vi "Check for Target Crossing.vi"(7 "target value":dbl, 9 "previous value":dbl, 11 "current value":dbl) -> (3 "crossed":bool)   [LabVIEW 2022 SP3]
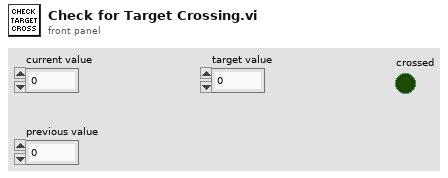
[diagram p1: front panel]
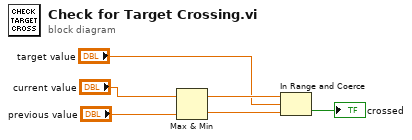
[diagram p0: block diagram]
diagram:
  n1 = Max & Min(x="current value", y="previous value") -> (max(x,y)=w6:dbl, min(x,y)=w5:dbl)
  n2 = In Range and Coerce(upper limit=w6, x="target value", lower limit=w5) -> (In Range?=→"crossed":bool)  [unwired: 1 out]
